vi "HEWH_Alicat_GasMeter.vi"(8 "error in":errorcluster, 11 "Message Queues out":T4) -> (0 "error out":errorcluster)   [LabVIEW 2023]
uses:
  Tenney/support/Message Queue/All Message Queues.ctl
  Tenney/support/Message Queue/Message Cluster.ctl
  Type Definitions/Alicat Gas Meter Data.ctl
  Drivers/Alicat Gas Meter Driver/Sub-VIs/Data Cluster.ctl
  Drivers/Alicat Gas Meter Driver/Sub-VIs/Units of Measure.ctl
  Drivers/Omega FMA-1600A Series Gas Flow Meter/Type Definitions/FMA1600A Gas Type.ctl
  FVIR and LDO/support/Message Queue/Enqueue Message (Single).vi
  FVIR and LDO/support/Message Queue/Message Queue.lvlib
  Tenney/support/Message Queue/Tenney Message Queue.lvlib
panel:
  out "Loop Count":i32
  out "output cluster":T1
  in  "Debug":bool
  out "Debug":string[](array[string])
  # "Totalizer Timer"
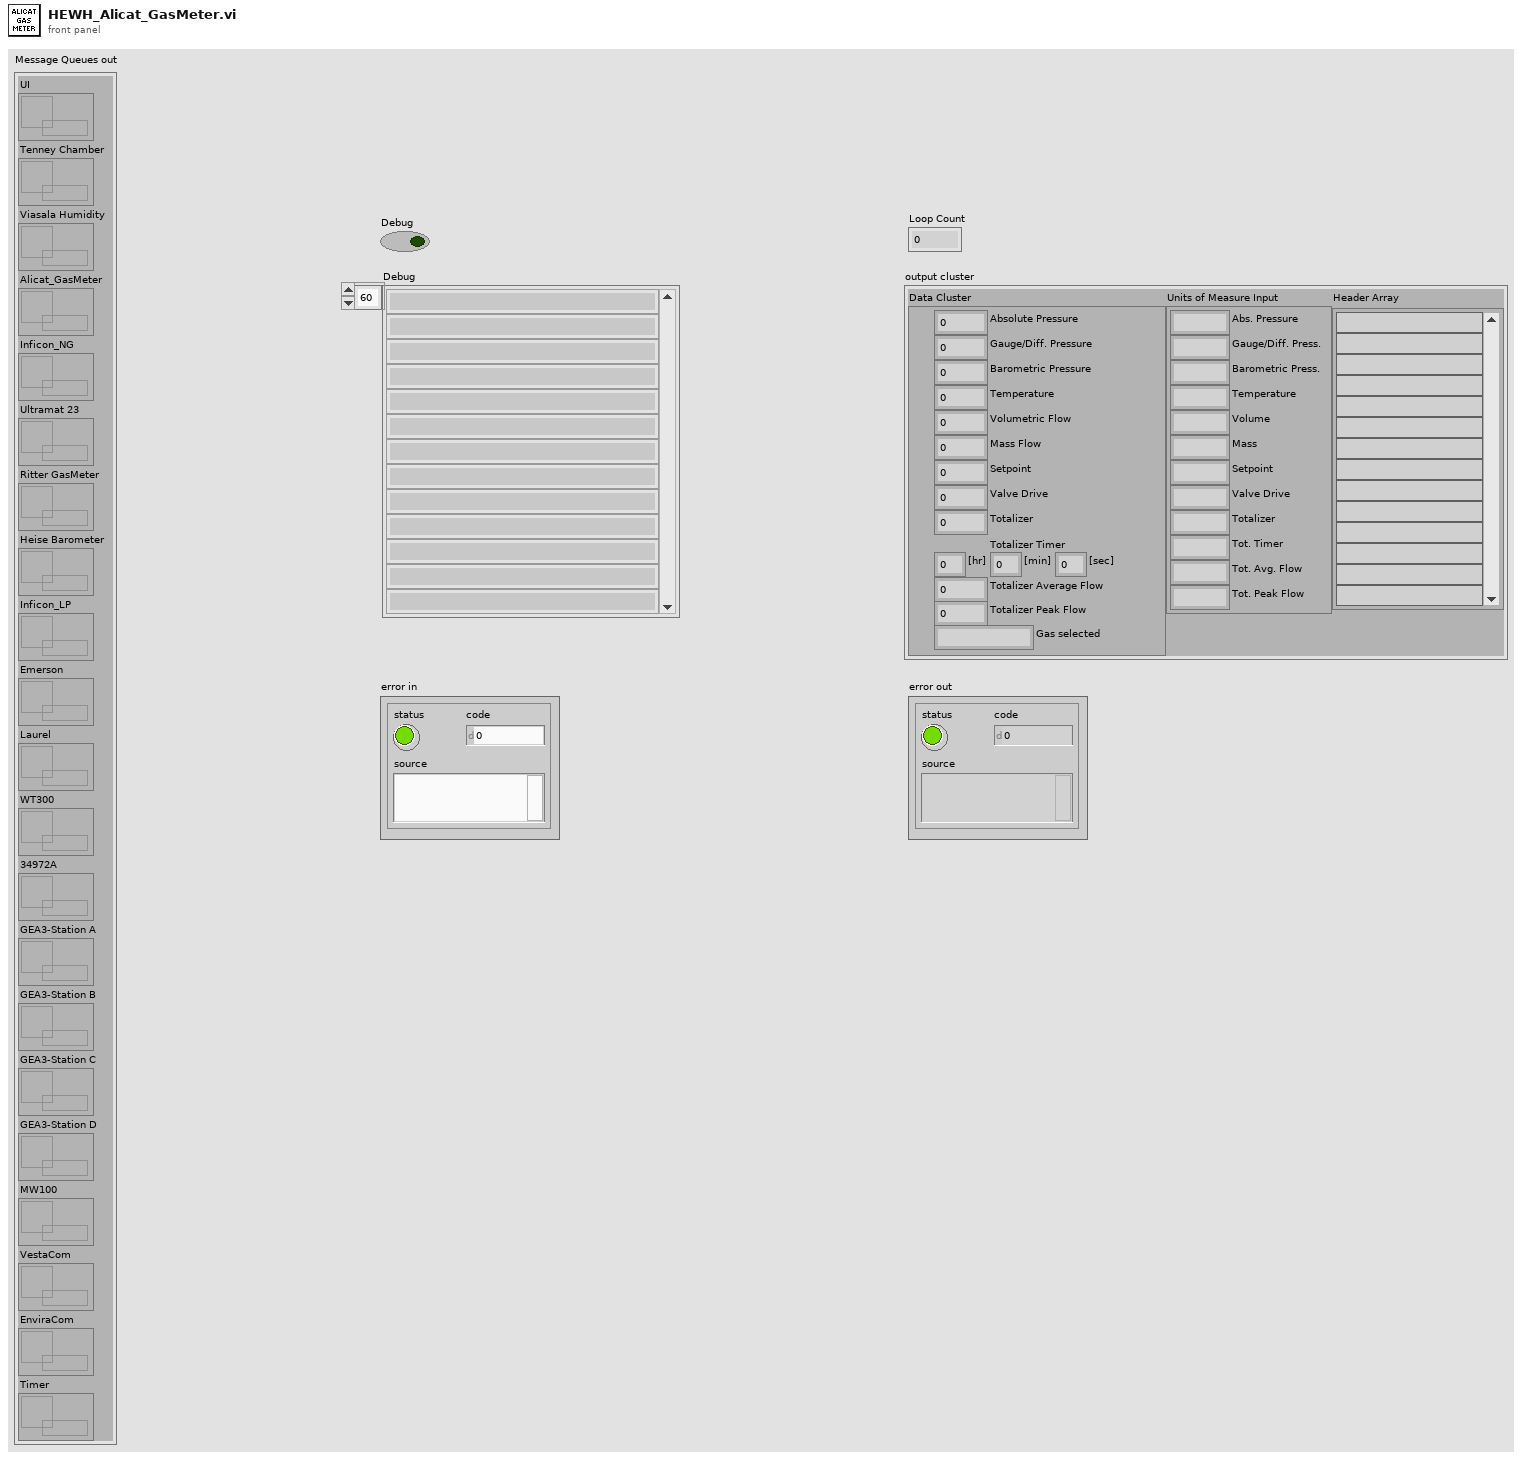
[diagram p1: front panel]
types:
  T1 = typedef "Alicat Gas Meter Data.ctl" = cluster{"Data Cluster":T2, "Units of Measure Input":T3, "Header Array":string[]}
  T2 = typedef "Data Cluster.ctl" = cluster{"Absolute Pressure":dbl, "Gauge/Diff. Pressure":dbl, "Barometric Pressure":dbl, "Temperature":dbl, "Volumetric Flow":dbl, "Mass Flow":dbl, "Setpoint":dbl, "Valve Drive":dbl, "Totalizer":dbl, "[hr]":dbl, "[min]":dbl, "[sec]":dbl, "Totalizer Average Flow":dbl, "Totalizer Peak Flow":dbl, "Gas selected":string}
  T3 = typedef "Units of Measure.ctl" = cluster{"Abs. Pressure":string, "Gauge/Diff. Press.":string, "Barometric Press.":string, "Temperature":string, "Volume":string, "Mass":string, "Setpoint":string, "Valve Drive":string, "Totalizer":string, "Tot. Timer":string, "Tot. Avg. Flow":string, "Tot. Peak Flow":string}
  T4 = typedef "Tenney Message Queue.lvlib/All Message Queues.ctl" = cluster{"UI":refnum<queue>, "Tenney Chamber":refnum<queue>, "Viasala Humidity":refnum<queue>, "Alicat_GasMeter":refnum<queue>, "Inficon_NG":refnum<queue>, "Ultramat 23":refnum<queue>, "Ritter GasMeter":refnum<queue>, "Heise Barometer":refnum<queue>, "Inficon_LP":refnum<queue>, "Emerson":refnum<queue>, "Laurel":refnum<queue>, "WT300":refnum<queue>, "34972A":refnum<queue>, "GEA3-Station A":refnum<queue>, "GEA3-Station B":refnum<queue>, "GEA3-Station C":refnum<queue>, "GEA3-Station D":refnum<queue>, "MW100":refnum<queue>, "VestaCom":refnum<queue>, "EnviraCom":refnum<queue>, "Timer":refnum<queue>}
  T5 = cluster{"Absolute Press.":bool, "Gauge/Diff. Press.":bool, "Barometric Press.":bool, "Temperature":bool, "Volumetric":bool, "Mass Flow":bool, "Setpoint":bool, "Valve Drive":bool, "Totalizer":bool, "Tot. Timer [s]":bool, "Tot. Avg. Flow":bool, "Tot. Peak Flow":bool, "Gas Selected":bool, "Log Data":bool}
  T6 = typedef "FMA1600A Gas Type.ctl" = string
  T7 = typedef "Data Frame.ctl" = cluster{"Absolute Pressure":bool, "Gauge/Diff. Pressure":bool, "Barometric Pressure":bool, "Temperature":bool, "Volumetric":bool, "Mass":bool, "Setpoint":bool, "Valve Drive":bool, "Totalizer":bool, "Totalizer Timer":bool, "Totalizer Average Flow":bool, "Totalizer Peak Flow":bool, "Gas Selected":bool, "Tot. Timer Format":u16}
  T8 = typedef "FMA1600A Units String.ctl" = cluster{"Software Rev":string, "Model Number":string, "Manufacturer Info":string, "Software Sub-Rev":string, "Board Rev":string, "Units of Measure Input":T3}
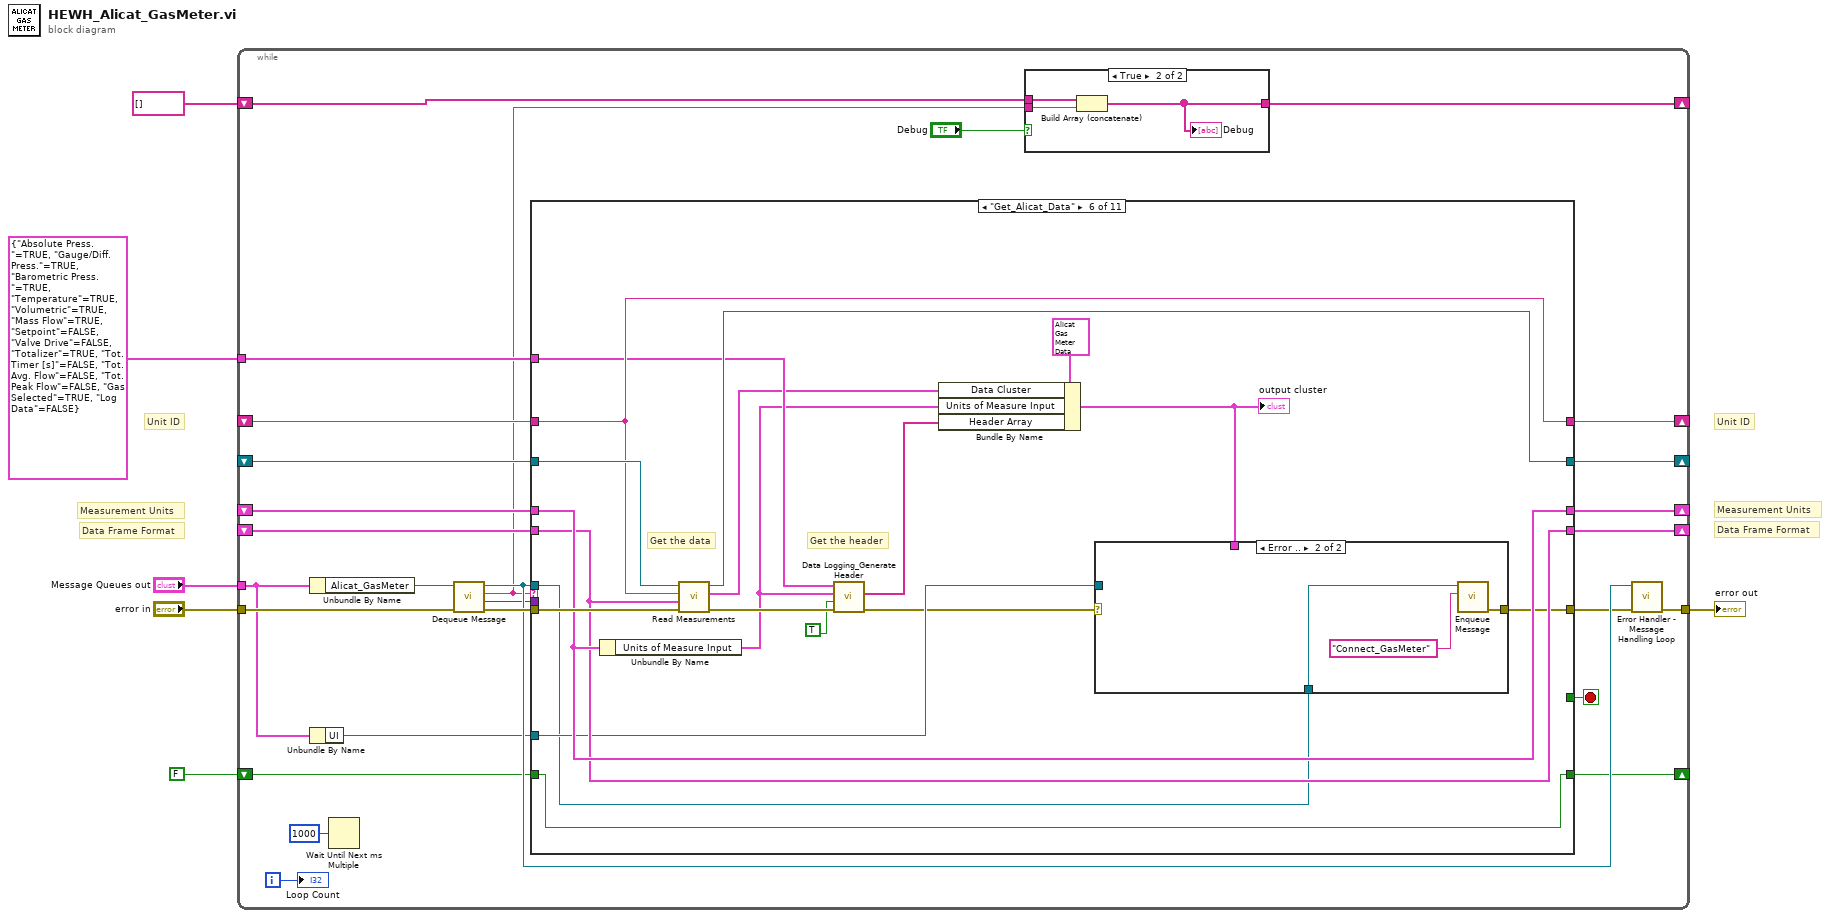
[diagram p0: block diagram]
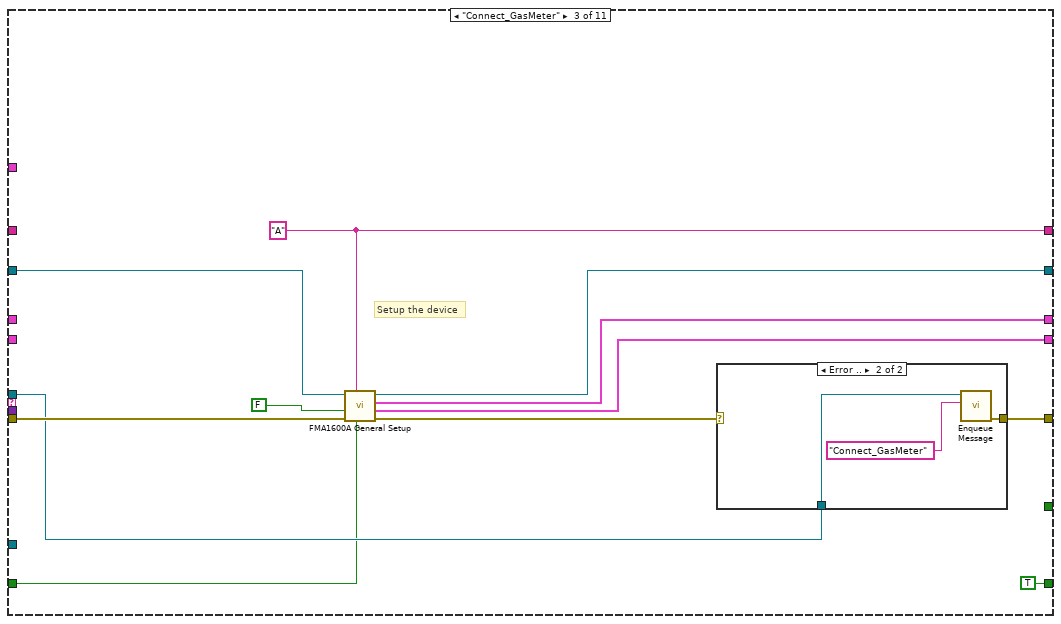
[diagram p5: hidden frame]
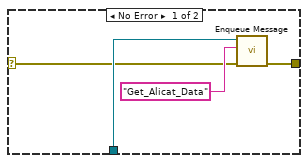
[diagram p6: hidden frame]
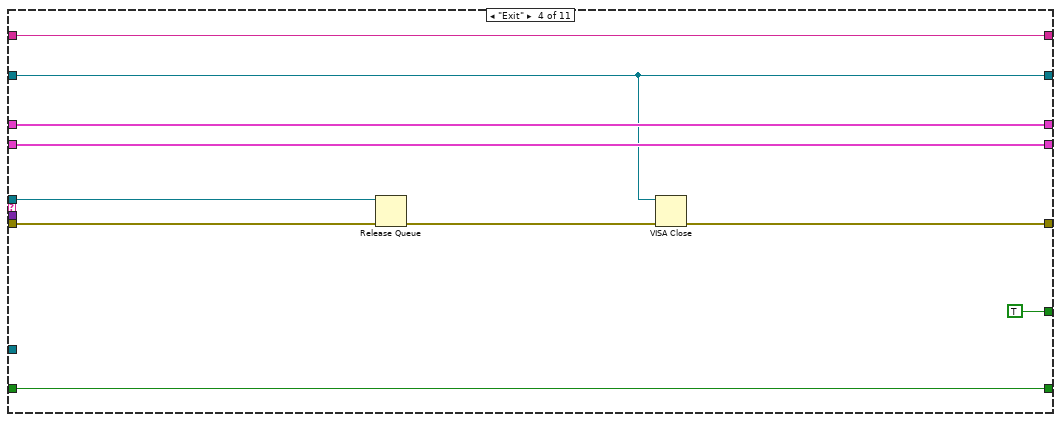
[diagram p7: hidden frame]
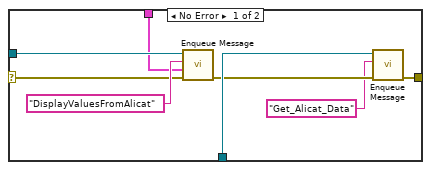
[diagram p9: hidden frame]
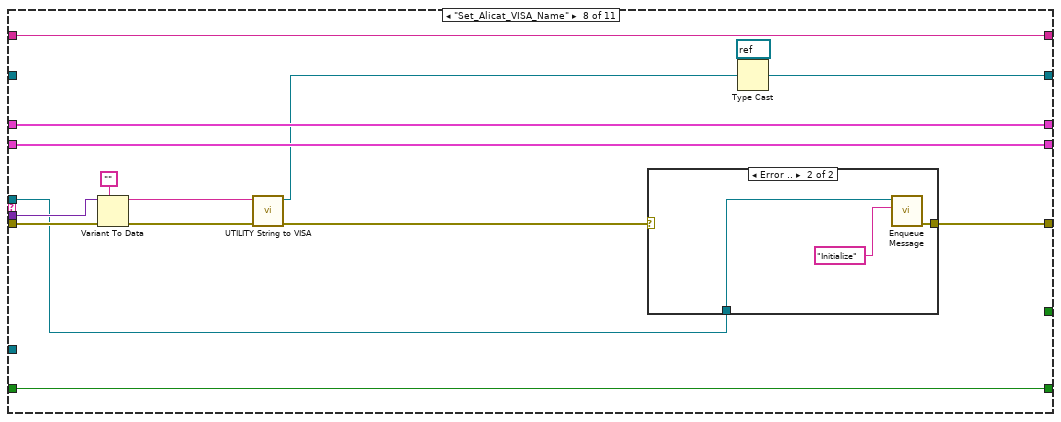
[diagram p11: hidden frame]
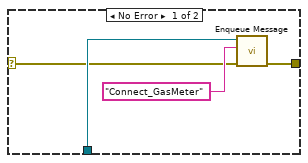
[diagram p12: hidden frame]
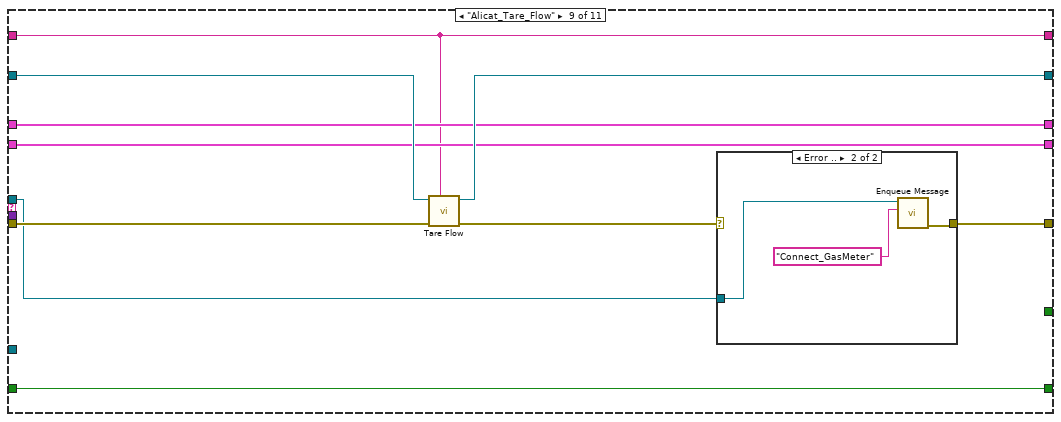
[diagram p13: hidden frame]
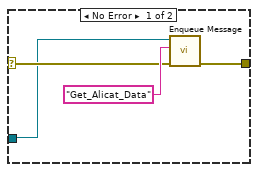
[diagram p14: hidden frame]
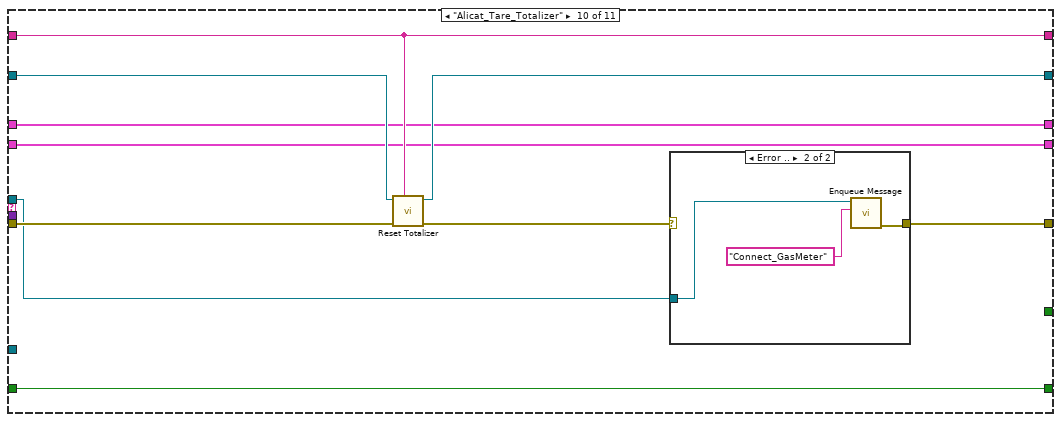
[diagram p15: hidden frame]
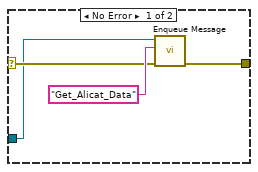
[diagram p16: hidden frame]
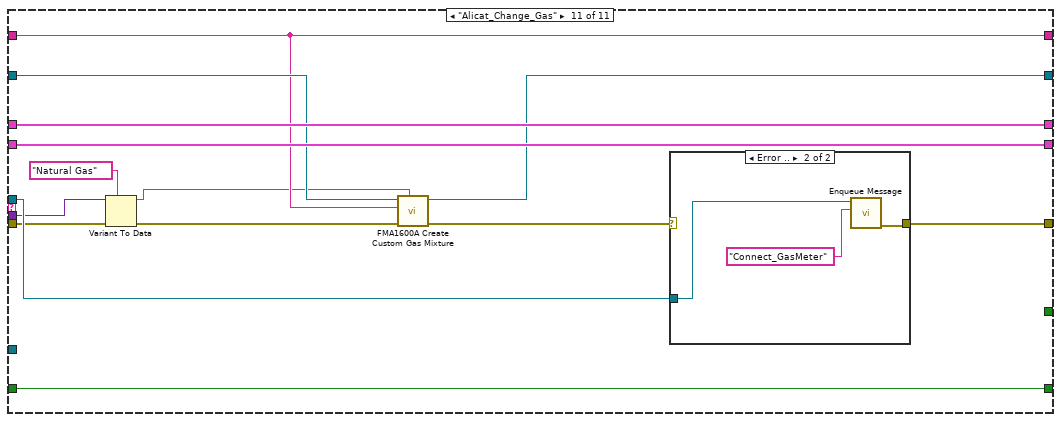
[diagram p17: hidden frame]
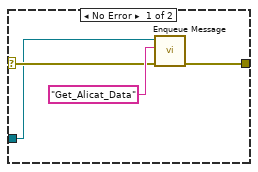
[diagram p18: hidden frame]
diagram:
  # "Unit ID"
  # "Data Frame Format"
  # "Measurement Units"
  # "Unit ID"
  # "Data Frame Format"
  # "Measurement Units"
  n1 = while {
    tunnel: "Message Queues out" -> [w16]
    tunnel: "error in" -> [w32]
    tunnel: [w28] -> w5
    shift-right: [w26] -> _
    shift-left: _ -> [w25]
    shift-right: [w23] -> _
    shift-left: _ -> [w20]
    shift-right: [w22] -> _
    shift-left: _ -> [w21]
    shift-right: [w19] -> _
    shift-left: _ -> [w18]
    tunnel: T5 {"Absolute Press."=TRUE, "Gauge/Diff. Press."=TRUE, "Barometric Press."=TRUE, "Temperature"=TRUE, "Volumetric"=TRUE, "Mass Flow"=TRUE, "Setpoint"=FALSE, "Valve Drive"=FALSE, "Totalizer"=TRUE, "Tot. Timer [s]"=FALSE, "Tot. Avg. Flow"=FALSE, "Tot. Peak Flow"=FALSE, "Gas Selected"=TRUE, "Log Data"=FALSE} ("Data Logging Options") -> [w17]
    shift-right: [w12] -> _
    shift-left: string[] [] -> [w13]
    shift-right: [w9] -> _
    shift-left: FALSE -> [w10]
    i -> [w7]
    stop <- w30 stop-if-true
    n2 = Unbundle By Name(w16) -> ("Alicat_GasMeter"=w33:refnum<queue>)
    n3 = Unbundle By Name(w16) -> ("UI"=w15:refnum<queue>)
    n4 = Wait Until Next ms Multiple(millisecond multiple=u32 1000) -> ()  [unwired: 1 out]
    n5 = call "Dequeue Message.vi"("error in (no error)"=w32, "Message Queue"=w33) -> ("error out"=w31:errorcluster, "Message Data"=w8:variant, "Message"=w14:string, "dup Message Queue"=w29:refnum<queue>)  [unwired: 6 in]
    n6 = case shown="\"Get_Alicat_Data\"" w14 {
      tunnel: w31 -> [w38 w44 w60 w69 w79 w100 w115 w130 w152 w169 w181]
      tunnel: [w38 w44 w56 w71 w79 w93 w115 w122 w143 w161 w187] -> w27
      tunnel: [_ _ _ TRUE _ _ _ _ _ _ _] -> w30
      tunnel: w29 -> [_ _ w55 w77 _ w92 _ w121 w144 w160 w186]
      tunnel: [w43 w49 w59 w70 w84 w101 w120 w124 w150 w166 w183] -> w26
      tunnel: w25 -> [w43 w49 w50 w70 w84 w99 w120 _ w151 w168 w184]
      tunnel: [w41 w47 w58 w75 w82 w97 w118 w134 w149 w165 w190] -> w23
      tunnel: [w40 w46 w57 w74 w81 w96 w117 w133 w148 w164 w189] -> w22
      tunnel: w21 -> [w40 w46 _ w74 w81 w96 w117 w133 w148 w164 w189]
      tunnel: w20 -> [w41 w47 _ w75 w82 w97 w118 w134 w149 w165 w190]
      tunnel: [w42 w48 w54 w76 w83 w98 w119 w135 w147 w167 w182] -> w19
      tunnel: w18 -> [w42 w48 _ w76 w83 w98 w119 w135 w147 w167 w182]
      tunnel: w17 -> [_ _ _ _ _ w95 _ _ _ _ _]
      tunnel: w15 -> [_ _ _ _ _ w94 _ _ _ _ _]
      tunnel: w10 -> [w39 w45 w52 w73 w80 w86 w116 w132 w146 w163 w188]
      tunnel: [w39 w45 TRUE w73 w80 w86 w116 w132 w146 w163 w188] -> w9
      tunnel: w8 -> [_ _ _ _ _ _ _ w129 _ _ w179]
      frame "---------- Setup ----------" {
      }
      frame "Initialize", Default {
      }
      frame "Connect_GasMeter" {
        w54 = "A" ("Unit ID")
        # "Setup the device"
        n7 = call "FMA1600A General Setup.vi"("Skip Dialog"=w52, "Unit ID"=w54, "error in (no error)"=w60, "Select Gas?"=FALSE, "VISA Refnum in"=w50) -> ("error out"=w51:errorcluster, "Data Frame Format"=w57:T7, "Measurement Units"=w58:T8, "VISA Refnum out"=w59:refnum<visa-resource-name>)  [unwired: 3 in]
        n8 = case shown="Error .." w51 {
          selector: w51 -> [w62 _]
          tunnel: [w64 w67] -> w56
          tunnel: w55 -> [w63 w66]
          frame No Error {
            n9 = call-poly "Enqueue Message.vi"("error in (no error)"=w62, "Message"="Get_Alicat_Data", "Message Queue"=w63) -> ("error out"=w64:errorcluster)  [unwired: 7 in, 1 out]
          }
          frame Error {
            n10 = call-poly "Enqueue Message.vi"("Message"="Connect_GasMeter", "Message Queue"=w66) -> ("error out"=w67:errorcluster)  [unwired: 8 in, 1 out]
          }
        }
      }
      frame "Exit" {
        n11 = Release Queue(queue=w77, error in (no error)=w69) -> (error out=w72:errorcluster)  [unwired: 1 in, 2 out]
        n12 = VISA Close(VISA resource name=w70, error in (no error)=w72) -> (error out=w71:errorcluster)
      }
      frame "---------- Data Collection ----------" {
      }
      frame "Get_Alicat_Data" {
        # "Get the header"
        # "Get the data"
        n13 = Unbundle By Name(w97) -> ("Units of Measure Input"=w89:T3)
        n14 = call "Read Measurements.vi"("error in"=w100, "Data Frame Format In"=w96, "Unit ID (A)"=w98, "VISA Session In"=w99) -> ("error out"=w103:errorcluster, "Data Cluster"=w90:T2, "VISA Session Out"=w101:refnum<visa-resource-name>)  [unwired: 5 out]
        n15 = call "Data Logging_Generate Header.vi"("error in"=w103, "Include Units\nin Header (F)"=TRUE ("Include Units\nin Header (default is F)"), "Units of Measure Input"=w89, "Data Logging Options"=w95) -> ("error out"=w85:errorcluster, "Header Array"=w88:string[])  [unwired: 5 in, 1 out]
        n16 = Bundle By Name(cluster=T1 {"Data Cluster"={"Absolute Pressure"=0.0, "Gauge/Diff. Pressure"=0.0, "Barometric Pressure"=0.0, "Temperature"=0.0, "Volumetric Flow"=0.0, "Mass Flow"=0.0, "Setpoint"=0.0, "Valve Drive"=0.0, "Totalizer"=0.0, "[hr]"=0.0, "[min]"=0.0, "[sec]"=0.0, "Totalizer Average Flow"=0.0, "Totalizer Peak Flow"=0.0, "Gas selected"=""}, "Units of Measure Input"={"Abs. Pressure"="", "Gauge/Diff. Press."="", "Barometric Press."="", "Temperature"="", "Volume"="", "Mass"="", "Setpoint"="", "Valve Drive"="", "Totalizer"="", "Tot. Timer"="", "Tot. Avg. Flow"="", "Tot. Peak Flow"=""}, "Header Array"=[]} ("Gas Data"), "Data Cluster"=w90, "Units of Measure Input"=w89, "Header Array"=w88) -> (w87:T1)
        "output cluster" <- w87
        n17 = case shown="Error .." w85 {
          selector: w85 -> [w104 _]
          tunnel: w94 -> [w110 _]
          tunnel: [w109 w113] -> w93
          tunnel: w92 -> [w108 w112]
          tunnel: w87 -> [w107 _]
          frame No Error {
            n18 = call-poly "Enqueue Message.vi"("error in (no error)"=w104, "Message Data"=w107, "Message"="DisplayValuesFromAlicat", "Message Queue"=w110) -> ("error out"=w106:errorcluster)  [unwired: 6 in, 1 out]
            n19 = call-poly "Enqueue Message.vi"("error in (no error)"=w106, "Message"="Get_Alicat_Data", "Message Queue"=w108) -> ("error out"=w109:errorcluster)  [unwired: 7 in, 1 out]
          }
          frame Error {
            n20 = call-poly "Enqueue Message.vi"("Message"="Connect_GasMeter", "Message Queue"=w112) -> ("error out"=w113:errorcluster)  [unwired: 8 in, 1 out]
          }
        }
      }
      frame "---------- Event ----------" {
      }
      frame "Set_Alicat_VISA_Name" {
        n21 = Variant To Data(error in=w130, type="", Variant=w129) -> (data=w127:string, error out=w128:errorcluster)
        n22 = call "UTILITY String to VISA.vi"("error in (no error)"=w128, "VISA Name"=w127) -> ("error out"=w123:errorcluster, "VISA resource name out"=w126:refnum<visa-resource-name>)  [unwired: 8 in]
        n23 = case shown="Error .." w123 {
          selector: w123 -> [w136 _]
          tunnel: [w138 w141] -> w122
          tunnel: w121 -> [w137 w140]
          frame No Error {
            n24 = call-poly "Enqueue Message.vi"("error in (no error)"=w136, "Message"="Connect_GasMeter", "Message Queue"=w137) -> ("error out"=w138:errorcluster)  [unwired: 7 in, 1 out]
          }
          frame Error {
            n25 = call-poly "Enqueue Message.vi"("Message"="Initialize", "Message Queue"=w140) -> ("error out"=w141:errorcluster)  [unwired: 8 in, 1 out]
          }
        }
        n26 = Type Cast(type=refnum<visa-resource-name> refnum ("VISA Refnum out"), x=w126) -> (*(type *) &x=w124:refnum<visa-resource-name>)
      }
      frame "Alicat_Tare_Flow" {
        n27 = call "Tare Flow.vi"("Unit ID (A)"=w147, "error in"=w152, "VISA Session In"=w151) -> ("error out"=w145:errorcluster, "VISA Session Out"=w150:refnum<visa-resource-name>)  [unwired: 7 in]
        n28 = case shown="Error .." w145 {
          selector: w145 -> [w155 _]
          tunnel: w144 -> [w153 w158]
          tunnel: [w154 w157] -> w143
          frame No Error {
            n29 = call-poly "Enqueue Message.vi"("error in (no error)"=w155, "Message"="Get_Alicat_Data", "Message Queue"=w153) -> ("error out"=w154:errorcluster)  [unwired: 7 in, 1 out]
          }
          frame Error {
            n30 = call-poly "Enqueue Message.vi"("Message"="Connect_GasMeter", "Message Queue"=w158) -> ("error out"=w157:errorcluster)  [unwired: 8 in, 1 out]
          }
        }
      }
      frame "Alicat_Tare_Totalizer" {
        n31 = call "Reset Totalizer.vi"("Unit ID (A)"=w167, "error in"=w169, "VISA Session In"=w168) -> ("error out"=w162:errorcluster, "VISA Session Out"=w166:refnum<visa-resource-name>)  [unwired: 6 in, 1 out]
        n32 = case shown="Error .." w162 {
          selector: w162 -> [w171 _]
          tunnel: w160 -> [w170 w175]
          tunnel: [w172 w174] -> w161
          frame No Error {
            n33 = call-poly "Enqueue Message.vi"("error in (no error)"=w171, "Message"="Get_Alicat_Data", "Message Queue"=w170) -> ("error out"=w172:errorcluster)  [unwired: 7 in, 1 out]
          }
          frame Error {
            n34 = call-poly "Enqueue Message.vi"("Message"="Connect_GasMeter", "Message Queue"=w175) -> ("error out"=w174:errorcluster)  [unwired: 8 in, 1 out]
          }
        }
      }
      frame "Alicat_Change_Gas" {
        n35 = Variant To Data(error in=w181, type=T6 "Natural Gas" ("Gas Type 2"), Variant=w179) -> (data=w177:T6, error out=w180:errorcluster)
        n36 = call "FMA1600A Create Custom Gas Mixture.vi"("Gas Type"=w177, "Error In"=w180, "Unit ID"=w182, "VISA Refnum in"=w184) -> ("Error Out"=w185:errorcluster, "VISA Refnum out"=w183:refnum<visa-resource-name>)  [unwired: 6 in]
        n37 = case shown="Error .." w185 {
          selector: w185 -> [w192 _]
          tunnel: w186 -> [w191 w196]
          tunnel: [w193 w195] -> w187
          frame No Error {
            n38 = call-poly "Enqueue Message.vi"("error in (no error)"=w192, "Message"="Get_Alicat_Data", "Message Queue"=w191) -> ("error out"=w193:errorcluster)  [unwired: 7 in, 1 out]
          }
          frame Error {
            n39 = call-poly "Enqueue Message.vi"("Message"="Connect_GasMeter", "Message Queue"=w196) -> ("error out"=w195:errorcluster)  [unwired: 8 in, 1 out]
          }
        }
      }
    }
    n40 = case shown="True" "Debug" {
      tunnel: w14 -> [_ w37]
      tunnel: w13 -> [w34 w36]
      tunnel: [w34 w35] -> w12
      frame False {
      }
      frame True {
        n41 = Build Array (concatenate)(w36, w37) -> (w35:string[])
        "Debug" <- w35
      }
    }
    n42 = call "Error Handler - Message Handling Loop.vi"("error in (no error)"=w27, "Message Queue"=w29) -> ("dup error in"=w28:errorcluster)  [unwired: 8 in, 1 out]
    "Loop Count" <- w7
  }
  "error out" <- w5
